vi "Servo.vi"() -> ()   [LabVIEW 2012]
uses:
  <vilib>/rvi/eio/common/nirviEmuTemplateMethod_errors.vi
  <vilib>/eio/EIONode/EIONode.xnode
panel:
  in  "servo 2":u32=1500
  in  "Count(uSec) 2":u32=5000
  in  "servo 1":u32=1500
  in  "Count(uSec) 1":u32=5000
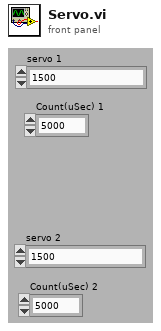
[diagram p1: front panel]
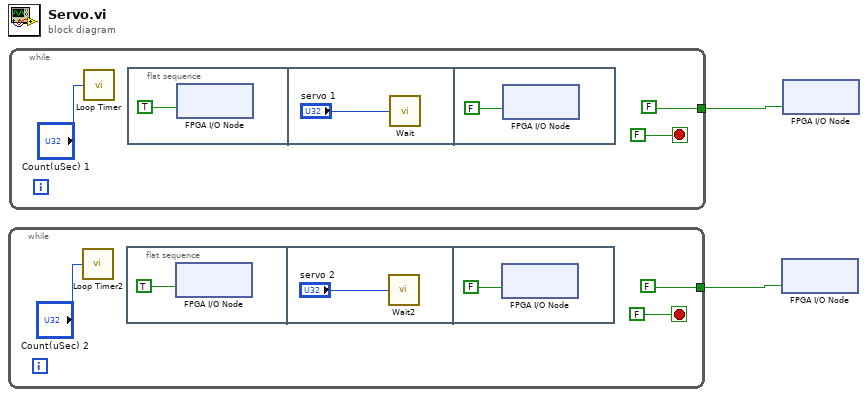
[diagram p0: block diagram]
diagram:
  n1 = while {
    tunnel: [FALSE ("Mod1/DO0")] -> w1
    stop <- FALSE stop-if-true
    n2 = call "Loop Timer2"("Count(uSec)"="Count(uSec) 2") -> ()  [unwired: 1 out]
    n3 = flat-sequence {
      frame #0 {
        n4 = xnode "FPGA I/O Node"("DIO1"=TRUE) -> ()  [unwired: 1 in, 1 out]
      }
      frame #1 {
        n5 = call "Wait2"("Count(uSec)"="servo 2") -> ()  [unwired: 1 out]
      }
      frame #2 {
        n6 = xnode "FPGA I/O Node"("DIO1"=FALSE) -> ()  [unwired: 1 in, 1 out]
      }
    }
  }
  n7 = while {
    tunnel: [FALSE ("Mod1/DO0")] -> w2
    stop <- FALSE stop-if-true
    n8 = call "Loop Timer"("Count(uSec)"="Count(uSec) 1") -> ()  [unwired: 1 out]
    n9 = flat-sequence {
      frame #0 {
        n10 = xnode "FPGA I/O Node"("DIO0"=TRUE) -> ()  [unwired: 1 in, 1 out]
      }
      frame #1 {
        n11 = call "Wait"("Count(uSec)"="servo 1") -> ()  [unwired: 1 out]
      }
      frame #2 {
        n12 = xnode "FPGA I/O Node"("DIO0"=FALSE) -> ()  [unwired: 1 in, 1 out]
      }
    }
  }
  n13 = xnode "FPGA I/O Node"("DIO1"=w1) -> ()  [unwired: 1 in, 1 out]
  n14 = xnode "FPGA I/O Node"("DIO0"=w2) -> ()  [unwired: 1 in, 1 out]
